vi "Check Variant Attributes.vi"(8 "error in (no error)":errorcluster, 11 "Dot Settings in":refnum<class "Dot Settings.lvclass">) -> (0 "error out":errorcluster, 3 "Dot Settings out":refnum<class "Dot Settings.lvclass">)   [LabVIEW 2019, in "Dot Settings.lvclass"]
uses:
  Dot Settings.lvclass
  TypeDefs/IV Settings.ctl
  Dot Settings.lvclass/Dot Settings.ctl
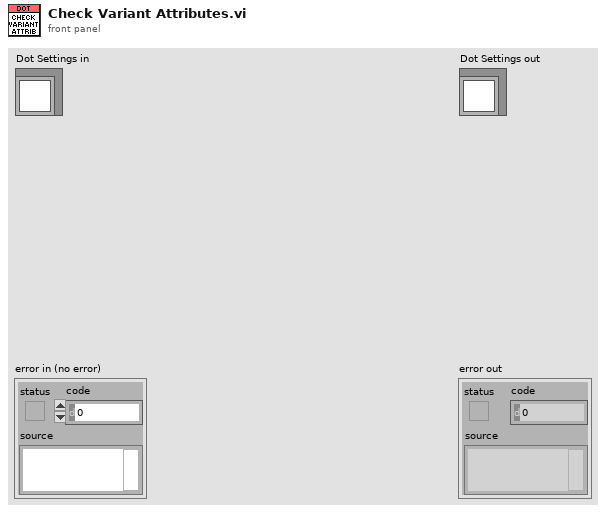
[diagram p1: front panel]
types:
  T1 = typedef "Dot Settings.lvclass/IV Settings.ctl" = cluster{"Pattern":enum16{"Ramp /", "Ramp /\\", "Smooth Ramp _/", "Smooth Ramp _/\\_", "Frequency"}, "Cycles":i32, "Rate":dbl, "End":dbl, "Start":dbl, "Port":u32, "Time":dbl, "Points":dbl[]}
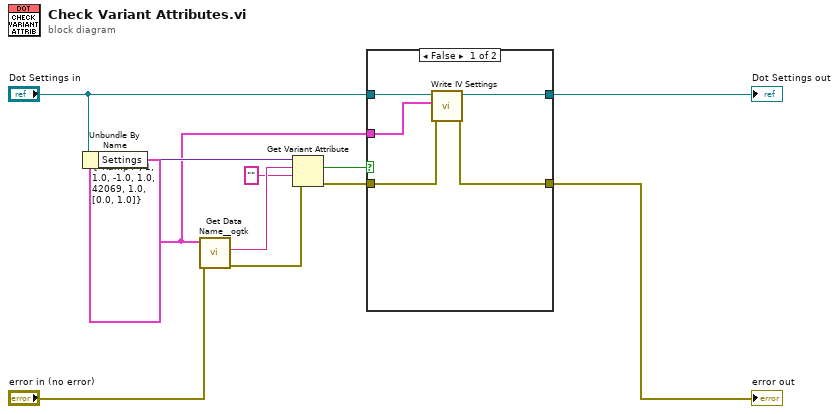
[diagram p0: block diagram]
diagram:
  w6 = T1 {"Pattern"=enum."Ramp /", "Cycles"=1, "Rate"=1.0, "End"=-1.0, "Start"=1.0, "Port"=42069, "Time"=1.0, "Points"=[0.0, 1.0]} ("IV Settings")
  n1 = Unbundle By Name("Dot Settings in") -> ("Settings"=w9:variant)
  n2 = call <userlib>:"Get Data Name__ogtk.vi"("error in (no error)"="error in (no error)", "Data"=w6) -> ("error out"=w4:errorcluster, "Data Name"=w11:string)  [unwired: 7 in, 1 out]
  n3 = Get Variant Attribute(Variant=w9, name=w11, default value (empty Variant)="", error in=w4) -> (found=w8:bool, error out=w3:errorcluster)  [unwired: 2 out]
  n4 = case shown="False" w8 {
    tunnel: "Dot Settings in" -> [w16 w18]
    tunnel: w6 -> [w15 _]
    tunnel: [w14 w18] -> w5
    tunnel: w3 -> [w13 w17]
    tunnel: [w12 w17] -> w1
    frame False {
      n5 = call "Write IV Settings.vi"("error in (no error)"=w13, "IV Settings"=w15, "Dot Settings in"=w16) -> ("error out"=w12:errorcluster, "Dot Settings out"=w14:refnum<class "Dot Settings.lvclass">)  [unwired: 7 in]
    }
    frame True {
    }
  }
  "error out" <- w1
  "Dot Settings out" <- w5
